vi "AODO-Create Tasks (DO).vi"(0 "DO":T1, 5 "DAQmx Device Name":tag, 11 "error in":errorcluster) -> (4 "task out":refnum<k21>, 15 "error out":errorcluster)   [LabVIEW 2020]
uses:
  Typedefs/DO-Output Spec.ctl
  <vilib>/DAQmx/create/channels.llb/DAQmx Create Channel (DO-Digital Output).vi
  <vilib>/DAQmx/configure/timing.llb/DAQmx Timing (Sample Clock).vi
  <resource>/objmgr/daqmx.rc
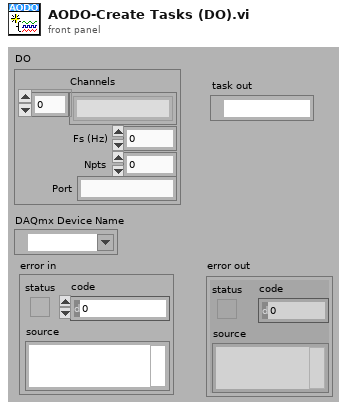
[diagram p1: front panel]
types:
  T1 = typedef "DO-Output Spec.ctl" = cluster{"Channels":string[], "Fs (Hz)":dbl, "Npts":i32, "Port":string}
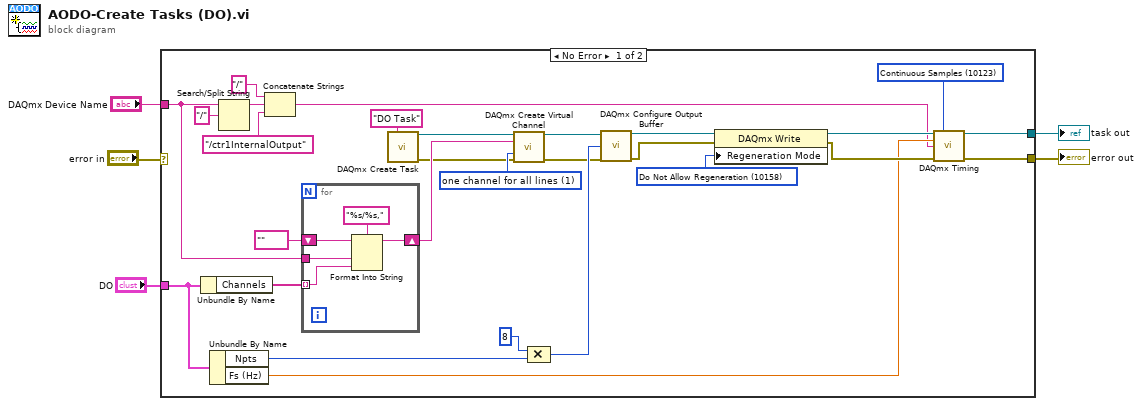
[diagram p0: block diagram]
diagram:
  n1 = case shown="No Error" "error in" {
    selector: "error in" -> [_ w39]
    tunnel: "DAQmx Device Name" -> [w12 _]
    tunnel: [w26 w39] -> w3
    tunnel: "DO" -> [w17 _]
    tunnel: [w14 _] -> w1
    frame No Error {
      w19 = 10158 items=["Allow Regeneration"=10097, "Do Not Allow Regeneration"=10158] ("RegenMode")
      w22 = 1 items=["one channel for each line", "one channel for all lines"] ("line grouping")
      w29 = 10123 items=["Finite Samples"=10178, "Continuous Samples"=10123, "Hardware Timed Single Point"=12522] ("sample mode")
      n2 = Unbundle By Name(w17) -> ("Channels"=w31:string[])
      n3 = Unbundle By Name(w17) -> ("Npts"=w15:i32, "Fs (Hz)"=w16:dbl)
      n4 = Search/Split String(string=w12, search string/char (-)="/") -> (substring before match=w11:string)  [unwired: 1 in, 2 out]
      n5 = Concatenate Strings("/", w11, "/ctr1InternalOutput") -> (w9:string)
      n6 = for {
        tunnel: w31 -> [w34] mode=indexing
        shift-right: [w36] -> w28
        shift-left: tag "" ("DAQmx Physical Channel") -> [w37]
        tunnel: w12 -> [w35]
        n7 = Format Into String(format string="%s/%s,", initial string=w37, w35, w34) -> (resulting string=w36:string)  [unwired: 1 in, 1 out]
      }
      n8 = call <vilib>:"DAQmx Create Task.vi"("new task name"="DO Task" ("name to assign")) -> ("task out"=w7:refnum<k21>, "error out"=w6:errorcluster)  [unwired: 13 in]
      n9 = call-poly <vilib>:"DAQmx Create Virtual Channel.vi"("task in"=w7, "lines"=w28, "line grouping"=w22, "error in"=w6) -> ("task out"=w21:refnum<k21>, "error out"=w20:errorcluster)  [unwired: 10 in]
      n10 = Compound Arithmetic op=MULTIPLY(8 ("x"), w15) -> (w23:i32)
      n11 = call <vilib>:"DAQmx Configure Output Buffer.vi"("task/channels in"=w21, "buffer size (in samples per channel)"=w23, "error in"=w20) -> ("task out"=w13:refnum<k21>, "error out"=w18:errorcluster)  [unwired: 11 in]
      n12 = property class="DAQmx Write"(reference=w13, error in=w18, "Regeneration Mode"=w19) -> (reference out=w24:refnum<k21>, error out=w25:errorcluster)
      n13 = call-poly <vilib>:"DAQmx Timing.vi"("task/channels in"=w24, "sample mode"=w29, "rate"=w16, "source"=w9, "error in"=w25) -> ("task out"=w14:refnum<k21>, "error out"=w26:errorcluster)  [unwired: 9 in]
    }
    frame Error {
    }
  }
  "error out" <- w3
  "task out" <- w1
